vi "TOOLweb Rezept wechseln.vi"() -> ()   [LabVIEW 2020, in "FT-IR.lvlib" / "TOOLweb Interface.lvlib"]
doc: "Holt mit einer HTTP-POST-Anforderung gemäß TOOLweb-Protokoll Messdaten, Einstellungen und Diagnose-Information vom MKS MultiGas 2030 Analyzer. Alle Daten werden zeitsparend in einem einzigen Poll Request zusammengefasst, damit nur einmal eine TCP/IP-Verbindung geöffnet werden muss.\n\nAlle Ergebnis-Datentypen sind als Typdefinitionen in der Bibliothek \"Datentypen\" enthalten\" und erlauben so eine spätere Erweiterung.\n\nFalls \"Anzahl Gase\" unverbunden bleibt, wird der Standardwert 18 verwendet.\n \nFalls der TOOLWeb-Server nicht auf demselben Rechner arbeitet, kann mit \"IP-Adresse\" eine beliebiger Host adressiert werden. Ein unverbundener Eingang spricht den lokalen Host an."
uses:
  TOOLweb Interface.lvlib
  Aktion Rezeptwechsel.ctl
  Aktion FGV Rezepte wechseln.ctl
  Aktionen EVID-Codes.ctl
  Trigger Aktionen.ctl
  Sprachverwaltung/FGV Aktion Tabelle zerlegen.ctl
  Funktionstasten/Freigabe Aktionen.ctl
  FGV FT-IR Diagnose Aktionen.ctl
  SysLog/SysLog Interface.ctl
  FGV FT-IR Aktionen.ctl
  Erweiterte Konfig/Konfig CG-Check/Aktion Aenderung bei Rezeptwechsel.ctl
  AK-Schnittstelle/AK Namen Aktionen.ctl
  FGV FT-IR Gasliste Aktionen.ctl
  Messdaten/Aktionen FGV Messdaten.ctl
  EPA 1065/Allgemeine VIs/Aktion Wertaenderung Gasliste.ctl
  Bildwechsel/Bild-Auswahl.ctl
  FT-IR.lvlib
  Allgemein/allgemeine Sub-VIs.lvlib
  Funktionstasten/Funktionstasten.lvlib
  Messdaten/Messdaten.lvlib
  Log Konfig/LogKonfig.lvlib
  Typdefinitionen.lvlib
  Bildwechsel/Bildwechsel.lvlib
  Erweiterte Konfig/Konfig CG-Check/CG-Check Konfig.lvlib
  AK interface/AK-Interface.lvlib
  AK interface/Kommandos verwalten Aktionen.ctl
  SysLog/SysLog.lvlib
  Sprachverwaltung/Sprachverwaltung.lvlib
  EPA 1065/EPA 1065.lvlib
  AK-Schnittstelle/AK-Schnittstelle.lvlib
panel:
  out "Feedback":i32
  out "reject code":string
  out "Status Rezept":string
  out "Neues Rezept":string
  # "Rezeptwechsel wird durchgeführt"
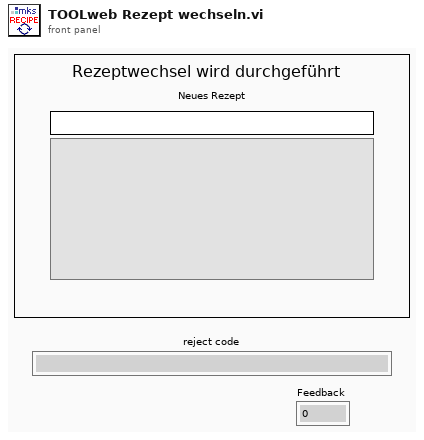
[diagram p1: front panel]
types:
  T1 = typedef "Sprachverwaltung.lvlib/FGV Aktion Tabelle zerlegen.ctl" = enum16{"laden", "vereinzeln", "speichern"}
  T2 = typedef "FT-IR.lvlib/TOOLweb Interface.lvlib/Typdefinitionen.lvlib/Trigger Aktionen.ctl" = enum16{"startrun", "runonce", "stoprun", "pauserun", "resumerun", "takeback"}
  T3 = typedef "FT-IR.lvlib/Aktionen EVID-Codes.ctl" = enum16{"lesen", "setzen", "laden", "speichern", "1Hz/5Hz", "Smoothing", "Rolling Average"}
  T4 = typedef "FT-IR.lvlib/Aktion FGV Rezepte wechseln.ctl" = enum16{"lesen", "Rezepte", "Rezeptindex", "Diesel", "Gasoline", "NCG", "laden", "speichern", "AK/Man"}
  T5 = typedef "FT-IR.lvlib/TOOLweb Interface.lvlib/Aktion Rezeptwechsel.ctl" = enum16{"Rezept wechsel", "Fehler", "Fehler 20", "Rezept geladen", "MG Bereit", "MG reagiert nicht", "Fertig", "Stoprun", "ueberpruefen"}
  T6 = typedef "Funktionstasten.lvlib/Freigabe Aktionen.ctl" = enum16{"prüfen", "Freigabe?", "lesen"}
  T7 = typedef "FT-IR.lvlib/AK-manuell.ctl" = enum16{"manuell", "Diesel", "CNG", "Gasoline"}
  T8 = typedef "FT-IR.lvlib/FGV FT-IR Diagnose Aktionen.ctl" = enum16{"Lesen", "Diagnose Schreiben", "Min Schreiben", "Max Schreiben"}
  T9 = cluster{"LaserPP Max":dbl, "LinCheck Max":dbl, "sBeam Max":dbl}
  T10 = cluster{"LaserPP Min":dbl, "LinCheck Min":dbl, "sBeam Min":dbl}
  T11 = typedef "FT-IR.lvlib/TOOLweb Interface.lvlib/Typdefinitionen.lvlib/TOOLweb Diagnose.ctl" = cluster{"(14) temperature":sgl, "(15) pressure":sgl, "(16) oxygen":sgl, "(50) diag-igramdc":sgl, "(51) diag-igrampp":sgl, "(52) diag-phaseAngle":sgl, "(53) diag-laserpp":sgl, "(54) diag-laserdc":sgl, "(55) diag-badscan":sgl, "(56) diag-centerburst":sgl, "(57) diag-linearizerCheck":sgl, "(58) diag-SNR":sgl, "(59) diag-sBeamIntensity":sgl}
  T12 = typedef "SysLog.lvlib/SysLog Interface.ctl" = cluster{"FehlermeldungsCode":i32, "ErfolgsmeldungsCode":i32, "ParameterListenString":string, "Anzeige":bool, "SysLogIcon":enum16{"OK", "Warnung", "Fehler"}, "intern":bool}
  T13 = typedef "FT-IR.lvlib/FGV FT-IR Aktionen.ctl" = enum16{"lesen", "NOG setzen", "NOS setzen", "Initialisieren", "speichern", "ALLES setzen", "FT-IR Spektrum loggen", "Komm Stoppen", "Spektrum LogKonfig"}
  T14 = typedef "AK-Schnittstelle.lvlib/AK Namen Aktionen.ctl" = enum16{"lesen", "laden", "speichern Namen", "AK Namen", "Liste erstellen", "EKFG erstellen", "speichern EKFG", "EKFG schreiben", "Neuen Eintrag erzeugen"}
  T15 = typedef "Erweiterte Konfig.lvlib/CG-Check Konfig.lvlib/Aktion Aenderung bei Rezeptwechsel.ctl" = enum16{"String erzeugen", "Index erzeugen"}
  T16 = typedef "FT-IR.lvlib/AK-Interface.lvlib/Kommandos verwalten Aktionen.ctl" = enum16{"lesen", "setzen Ende", "setzen Pos1", "senden", "initalisieren", "prüfen", "Kommandos"}
  T17 = typedef "FT-IR.lvlib/FGV FT-IR Gasliste Aktionen.ctl" = enum16{"lesen", "Gasliste FT-IR", "Gasliste ausgelesen", "laden", "speichern", "löschen"}
  T18 = typedef "Messdaten.lvlib/Aktionen FGV Messdaten.ctl" = enum16{"lesen", "schreiben", "löschen", "Mittelwerte", "Komponente"}
  T19 = typedef "EPA 1065.lvlib/Aktion Wertaenderung Gasliste.ctl" = enum16{"Init", "lesen", "Gasliste geändert", "ARN inaktiv", "LEAK inaktiv", "Interference 366 inaktiv", "T90 inaktiv", "Interference 375 inaktiv", "Chiller inaktiv", "FID O2 inaktiv", "FID Opti inaktiv", "Drift inaktiv", "Pre Test inaktiv", "LinV2 inaktiv"}
  T20 = typedef "Bildwechsel.lvlib/Bild-Auswahl.ctl" = enum16{"lesen", "Initialisieren", "Beenden", "Grafik", "Anlagenübersicht", "Anlagengrenzwerte", "Log Konfig", "Gaszuordnung AO", "Erw. Konfiguration", "FT-IR  ", "Störmeldungen", "Störmeldepuffer", "Störmeldekonfig", "PNS Grenzwerte", "Statusübersicht", "Linearisierung", "ARN", "EPA Dichtheitstest", "FID", "PMA", "CalGas", "Lambda", "Interference", "Amium PNS", "EPA T90", "Interference N2O", "Scheduler", "Systemeinstellungen", "EPA Drift", "CAN Konfig"}
  T21 = typedef "String - Ausgabefeld.ctl" = string
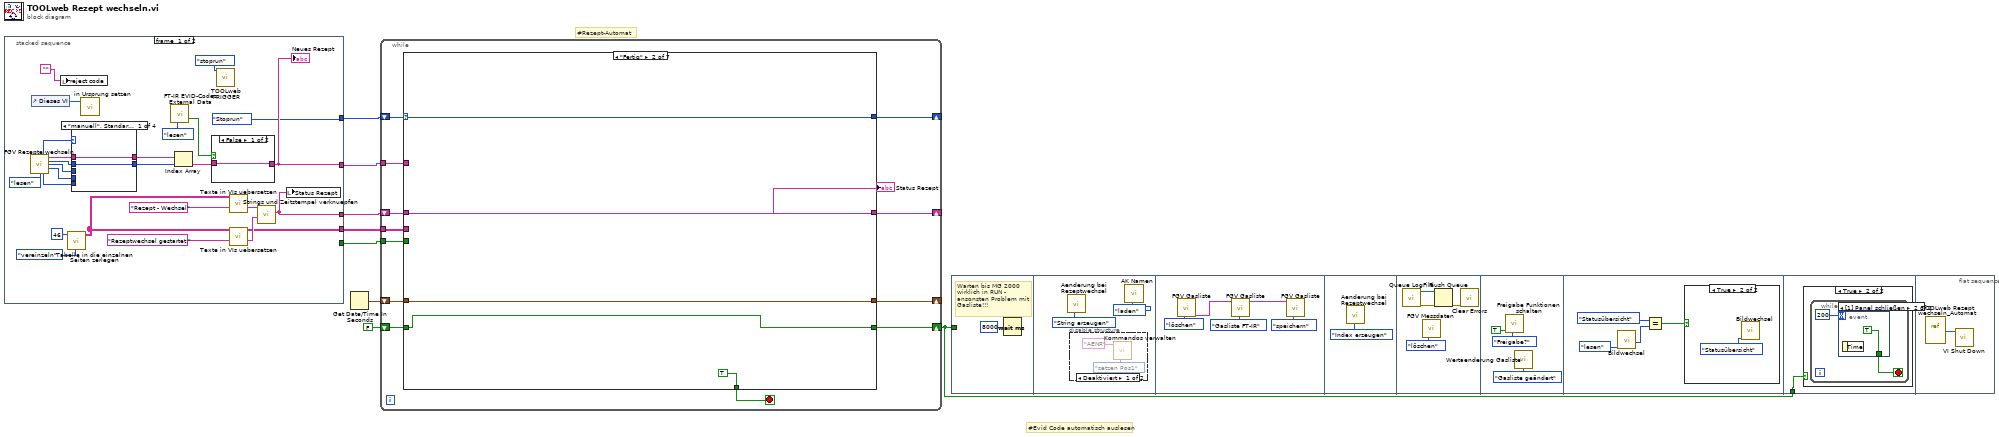
[diagram p0: block diagram]
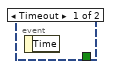
[diagram p5: hidden frame]
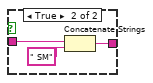
[diagram p6: hidden frame]
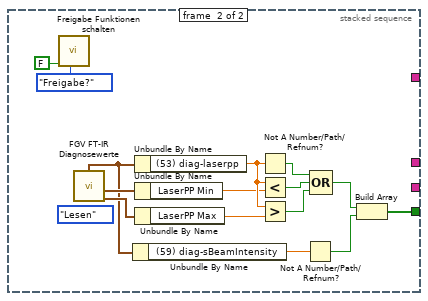
[diagram p10: hidden frame]
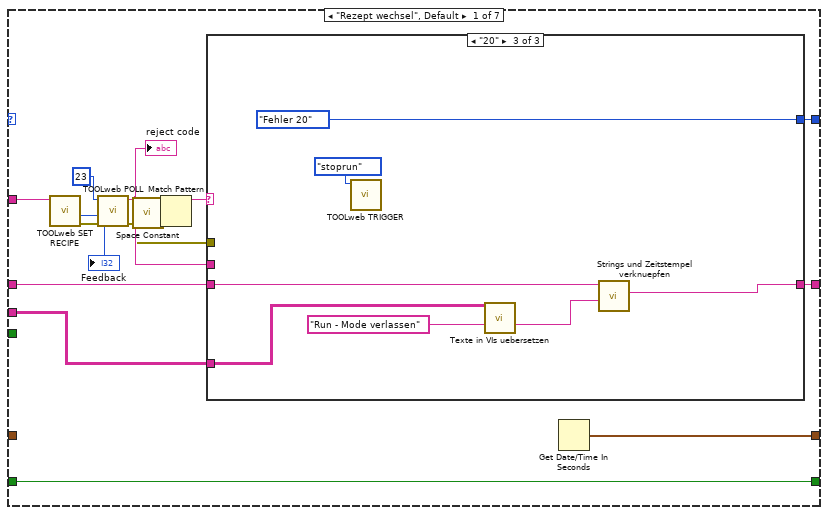
[diagram p11: hidden frame]
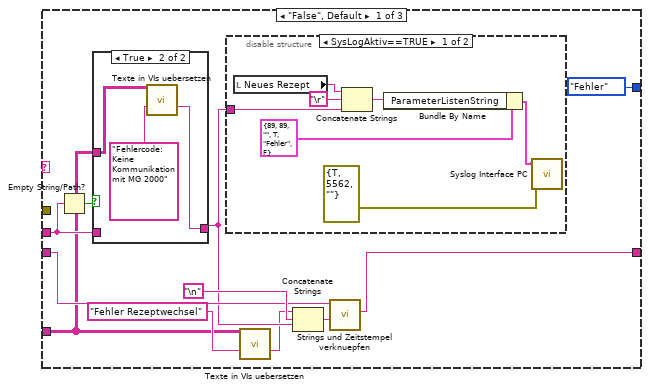
[diagram p12: hidden frame]
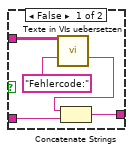
[diagram p14: hidden frame]
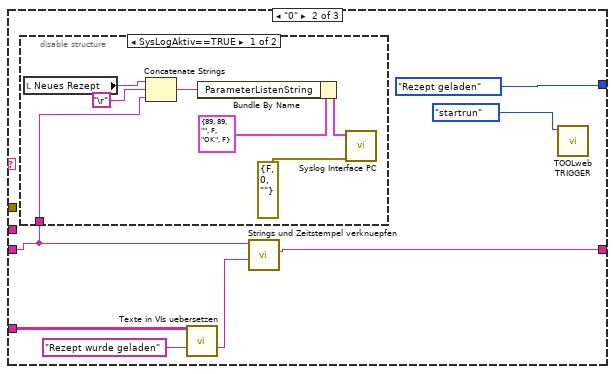
[diagram p15: hidden frame]
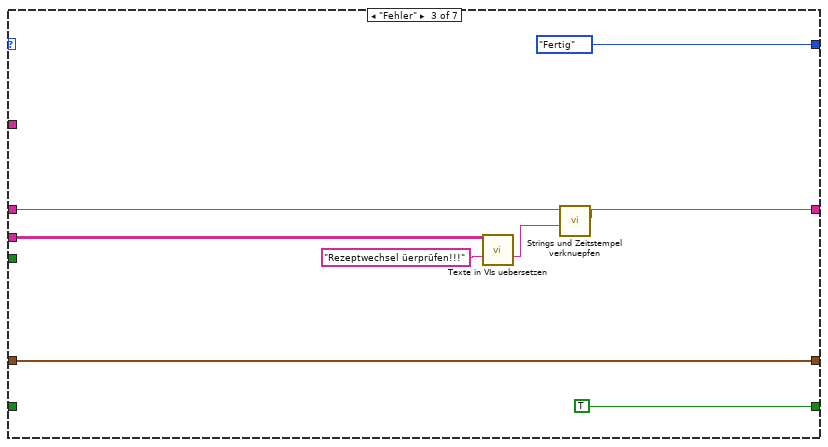
[diagram p17: hidden frame]
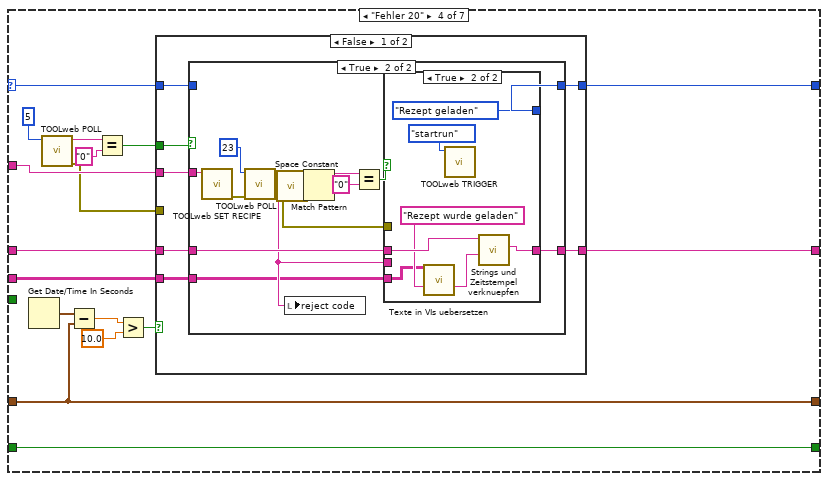
[diagram p18: hidden frame]
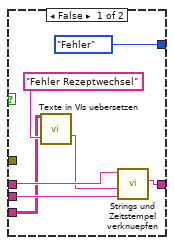
[diagram p20: hidden frame]
diagram:
  # "#Evid Code automatisch auslesen"
  # "#Rezept-Automat"
  n1 = stacked-sequence {
    tunnel: [w22 _] -> w8
    tunnel: [Aktion_Rezeptwechsel."Stoprun" ("Enum") _] -> w7
    tunnel: [w20 _] -> w6
    tunnel: [_ w47] -> w4
    tunnel: [w9 _] -> w1
    frame #0 {
      n2 = call "FGV Rezepte wechseln.vi"("Aktion"=Aktion_FGV_Rezepte_wechseln."lesen") -> ("AK/man"=w24:T7, "Rezepte"=w33:string[], "Rezeptindex"=w26:i32, "Diesel"=w28:u16, "Gasoline"=w29:u16, "Natural Gas"=w30:u16)  [unwired: 8 in, 1 out]
      n3 = control-ref of="Dieses VI"() -> (w18:refnum<vi>)
      n4 = local write "reject code"("") -> ()
      n5 = call "Tabelle in die einzelnen Seiten zerlegen.vi"("Aktion"=FGV_Aktion_Tabelle_zerlegen."vereinzeln", "Index (Seite)"=46) -> ("Sprachliste"=w10:string[][])  [unwired: 7 in, 2 out]
      n6 = case shown="\"manuell\", Standard" w24 {
        tunnel: w33 -> [w40 w42 w44 w45]
        tunnel: [w40 w42 w44 w45] -> w25
        tunnel: w26 -> [w39 _ _ _]
        tunnel: [w39 w41 w43 w46] -> w27
        tunnel: w28 -> [_ w41 _ _]
        tunnel: w29 -> [_ _ _ w46]
        tunnel: w30 -> [_ _ w43 _]
        frame "manuell", Default {
        }
        frame "Diesel" {
        }
        frame "CNG" {
        }
        frame "Gasoline" {
        }
      }
      n7 = call "in Ursprung setzen.vi"("VI Referenz"=w18) -> ()  [unwired: 10 in, 1 out]
      n8 = call "FT-IR EVID-Codes External Data.vi"("Aktionen"=Aktionen_EVID-Codes."lesen") -> ("Smoothing?"=w32:bool)  [unwired: 9 in, 5 out]
      n9 = Index Array(array=w25, index=w27) -> (element=w34:string)
      n10 = case shown="False" w32 {
        tunnel: w34 -> [w35 w37]
        tunnel: [w35 w38] -> w22
        frame False {
        }
        frame True {
          n11 = Concatenate Strings(w37, " SM" ("String")) -> (w38:string)
        }
      }
      "Neues Rezept" <- w22
      n12 = call "TOOLweb TRIGGER.vi"("action"=Trigger_Aktionen."stoprun") -> ()  [unwired: 5 in, 2 out]
      n13 = call "Texte in VIs uebersetzen.vi"("Sprachliste"=w10, "String zum Übersetzen"="Rezept - Wechsel") -> ("String zum Übersetzen"=w13:string)  [unwired: 9 in, 4 out]
      n14 = call "Texte in VIs uebersetzen.vi"("Sprachliste"=w10, "String zum Übersetzen"="Rezeptwechsel gestartet:") -> ("Sprachliste out"=w9:string[][], "String zum Übersetzen"=w11:string)  [unwired: 9 in, 3 out]
      n15 = call "Strings und Zeitstempel verknuepfen.vi"("String 1 hinzufügen"=w11, "Eingagns String"=w13) -> ("Verknüpfter String"=w20:string)  [unwired: 9 in]
      n16 = local write "Status Rezept"(w20) -> ()
    }
    frame #1 {
      (unwired) FGV_FT-IR_Diagnose_Aktionen."Lesen" ("Aktionen")
      n17 = call "Freigabe Funktionen schalten.vi"("Aktionen"=Freigabe_Aktionen."Freigabe?", "Freigabe?"=FALSE) -> ()  [unwired: 7 in, 3 out]
      n18 = call "FGV FT-IR Diagnosewerte.vi"() -> ("FT-IR MAX"=w58:T9, "FT-IR MIN"=w59:T10, "Diagnose"=w51:T11)  [unwired: 6 in, 3 out]
      n19 = Unbundle By Name(w51) -> ("(59) diag-sBeamIntensity"=w50:sgl)
      n20 = Unbundle By Name(w51) -> ("(53) diag-laserpp"=w57:sgl)
      n21 = Unbundle By Name(w59) -> ("LaserPP Min"=w56:dbl)
      n22 = Unbundle By Name(w58) -> ("LaserPP Max"=w55:dbl)
      n23 = Not A Number/Path/Refnum?(number/path/refnum=w57) -> (NaN/Path/Refnum?=w52:bool)
      n24 = Less?(x=w57, y=w56) -> (x < y?=w53:bool)
      n25 = Greater?(x=w57, y=w55) -> (0:w54:bool)
      n26 = Not A Number/Path/Refnum?(number/path/refnum=w50) -> (NaN/Path/Refnum?=w48:bool)
      n27 = Compound Arithmetic op=OR(w52, w53, w54) -> (w49:bool)
      n28 = Build Array(w49, w48) -> (w47:bool[])
    }
  }
  n29 = Get Date/Time In Seconds() -> (seconds since 1Jan1904=w2:timestamp)
  n30 = while {
    tunnel: w8 -> [w73]
    shift-right: [w72] -> _
    shift-left: w7 -> [w71]
    shift-right: [w70] -> _
    shift-left: w2 -> [w69]
    shift-right: [w65] -> _
    shift-left: w6 -> [w68]
    shift-right: [w66] -> w3
    shift-left: FALSE -> [w64]
    tunnel: w4 -> [w63]
    tunnel: w1 -> [w62]
    stop <- w67 stop-if-true
    n31 = case shown="\"Fertig\"" w71 {
      selector: w71 -> [_ w137 _ w153 w246 w285 _]
      tunnel: w73 -> [w87 _ _ w152 w245 w274 _]
      tunnel: [w82 w137 Aktion_Rezeptwechsel."Fertig" ("Enum") w160 w253 w286 Aktion_Rezeptwechsel."Fehler" ("Enum")] -> w72
      tunnel: w69 -> [_ w139 w146 w151 w244 w294 w329]
      tunnel: [w78 w139 w146 w151 w244 w294 w329] -> w70
      tunnel: w68 -> [w81 w138 w143 w159 w252 w282 w326]
      tunnel: [w80 w138 w144 w154 w247 w283 w328] -> w65
      tunnel: [_ TRUE _ _ _ _ _] -> w67
      tunnel: [w76 w135 TRUE w150 w243 w277 w327] -> w66
      tunnel: w64 -> [w76 w135 _ w150 w243 w277 w327]
      tunnel: w63 -> [_ _ _ _ _ _ _]
      tunnel: w62 -> [w74 _ w140 w148 _ w270 w323]
      frame "Rezept wechsel", Default {
        n32 = call "TOOLweb SET RECIPE.vi"("Recipe Name"=w87) -> ("error out"=w85:errorcluster, "Feedback"=→"Feedback":i32)  [unwired: 4 in, 1 out]
        n33 = call "TOOLweb POLL.vi"("error in (no error)"=w85, "EVID-Nummer"=23) -> ("error out"=w75:errorcluster, "Wert-String"=w79:string)  [unwired: 4 in]
        "reject code" <- w79
        n34 = call <vilib>:"Space Constant.vi"() -> ("String"=w84:string)
        n35 = Match Pattern(string=w79, regular expression=w84) -> (before substring=w83:string)  [unwired: 1 in, 3 out]
        n36 = case shown="\"20\"" w83 {
          tunnel: [Aktion_Rezeptwechsel."Fehler" ("Enum") Aktion_Rezeptwechsel."Rezept geladen" ("Enum") Aktion_Rezeptwechsel."Fehler 20" ("Enum")] -> w82
          tunnel: w81 -> [w95 w117 w131]
          tunnel: [w94 w119 w132] -> w80
          tunnel: w79 -> [w92 _ _]
          tunnel: w75 -> [_ _ _]
          tunnel: w74 -> [w88 w114 w128]
          frame "False", Default {
            n37 = Empty String/Path?(string/path=w92) -> (empty?=w93:bool)
            n38 = case shown="True" w93 {
              tunnel: [w110 w112] -> w91
              tunnel: w92 -> [w109 _]
              tunnel: w88 -> [w106 w111]
              frame False {
                n39 = call "Texte in VIs uebersetzen.vi"("Sprachliste"=w106, "String zum Übersetzen"="Fehlercode:" ("String")) -> ("String zum Übersetzen"=w107:string)  [unwired: 9 in, 4 out]
                n40 = Concatenate Strings(w107, w109) -> (w110:string)
              }
              frame True {
                n41 = call "Texte in VIs uebersetzen.vi"("Sprachliste"=w111, "String zum Übersetzen"="Fehlercode: Keine Kommunikation mit MG 2000" ("String")) -> ("String zum Übersetzen"=w112:string)  [unwired: 9 in, 4 out]
              }
            }
            n42 = disable-structure shown="SysLogAktiv==TRUE" {
              disable-tunnel: w91 -> [w102 _]
              frame condition #0 (active) {
                n43 = local read "Neues Rezept"() -> (w104:string)
                n44 = Concatenate Strings(w104, "\r", w102) -> (w99:string)
                n45 = Bundle By Name(cluster=T12 {"FehlermeldungsCode"=89, "ErfolgsmeldungsCode"=89, "ParameterListenString"="", "Anzeige"=TRUE, "SysLogIcon"=enum."Fehler", "intern"=FALSE} ("Cluster (in)"), "ParameterListenString"=w99) -> (w100:T12)
                n46 = call "Syslog Interface PC.vi"("Fehler (in)"=errorcluster {"status"=TRUE, "code"=5562, "source"=""}, "Cluster (in)"=w100) -> ()  [unwired: 9 in, 1 out]
              }
              frame condition #1 {
              }
            }
            n47 = call "Texte in VIs uebersetzen.vi"("Sprachliste"=w88, "String zum Übersetzen"="Fehler Rezeptwechsel" ("String")) -> ("String zum Übersetzen"=w89:string)  [unwired: 9 in, 4 out]
            n48 = Concatenate Strings(w89, "\n", w91) -> (w96:string)
            n49 = call "Strings und Zeitstempel verknuepfen.vi"("String 1 hinzufügen"=w96, "Eingagns String"=w95) -> ("Verknüpfter String"=w94:string)  [unwired: 9 in]
          }
          frame "0" {
            n50 = disable-structure shown="SysLogAktiv==TRUE" {
              disable-tunnel: w117 -> [w124 _]
              frame condition #0 (active) {
                n51 = local read "Neues Rezept"() -> (w126:string)
                n52 = Concatenate Strings(w126, "\r", w124) -> (w121:string)
                n53 = Bundle By Name(cluster=T12 {"FehlermeldungsCode"=89, "ErfolgsmeldungsCode"=89, "ParameterListenString"="", "Anzeige"=FALSE, "SysLogIcon"=enum."OK", "intern"=FALSE} ("Cluster (in)"), "ParameterListenString"=w121) -> (w122:T12)
                n54 = call "Syslog Interface PC.vi"("Fehler (in)"=errorcluster {"status"=FALSE, "code"=0, "source"=""}, "Cluster (in)"=w122) -> ()  [unwired: 9 in, 1 out]
              }
              frame condition #1 {
              }
            }
            n55 = call "Texte in VIs uebersetzen.vi"("Sprachliste"=w114, "String zum Übersetzen"="Rezept wurde geladen" ("String")) -> ("String zum Übersetzen"=w115:string)  [unwired: 9 in, 4 out]
            n56 = call "Strings und Zeitstempel verknuepfen.vi"("String 1 hinzufügen"=w115, "Eingagns String"=w117) -> ("Verknüpfter String"=w119:string)  [unwired: 9 in]
            n57 = call "TOOLweb TRIGGER.vi"("action"=Trigger_Aktionen."startrun") -> ()  [unwired: 5 in, 2 out]
          }
          frame "20" {
            n58 = call "TOOLweb TRIGGER.vi"("action"=Trigger_Aktionen."stoprun") -> ()  [unwired: 5 in, 2 out]
            n59 = call "Texte in VIs uebersetzen.vi"("Sprachliste"=w128, "String zum Übersetzen"="Run - Mode verlassen" ("String")) -> ("String zum Übersetzen"=w129:string)  [unwired: 9 in, 4 out]
            n60 = call "Strings und Zeitstempel verknuepfen.vi"("String 1 hinzufügen"=w129, "Eingagns String"=w131) -> ("Verknüpfter String"=w132:string)  [unwired: 9 in]
          }
        }
        n61 = Get Date/Time In Seconds() -> (seconds since 1Jan1904=w78:timestamp)
      }
      frame "Fertig" {
      }
      frame "Fehler" {
        n62 = call "Texte in VIs uebersetzen.vi"("Sprachliste"=w140, "String zum Übersetzen"="Rezeptwechsel üerprüfen!!!" ("String")) -> ("String zum Übersetzen"=w141:string)  [unwired: 9 in, 4 out]
        n63 = call "Strings und Zeitstempel verknuepfen.vi"("String 1 hinzufügen"=w141, "Eingagns String"=w143) -> ("Verknüpfter String"=w144:string)  [unwired: 9 in]
      }
      frame "Fehler 20" {
        n64 = Get Date/Time In Seconds() -> (seconds since 1Jan1904=w164:timestamp)
        n65 = call "TOOLweb POLL.vi"("EVID-Nummer"=5) -> ("error out"=w149:errorcluster, "Wert-String"=w157:string)  [unwired: 5 in]
        n66 = Subtract(x=w164, y=w151) -> (x-y=w163:dbl)
        n67 = Equal?(x=w157, y="0") -> (x = y?=w155:bool)
        n68 = Greater?(x=w163, y=10.0) -> (0:w161:bool)
        n69 = case shown="False" w161 {
          tunnel: [w170 w206] -> w160
          tunnel: w159 -> [w167 w204]
          tunnel: w155 -> [w171 w202]
          tunnel: [w168 w205] -> w154
          tunnel: w153 -> [w169 _]
          tunnel: w152 -> [w166 w203]
          tunnel: w149 -> [_ _]
          tunnel: w148 -> [w165 w201]
          frame False {
            n70 = case shown="True" w171 {
              tunnel: [w173 w179] -> w170
              tunnel: w169 -> [w173 _]
              tunnel: [w172 w177] -> w168
              tunnel: w167 -> [w172 w178]
              tunnel: w166 -> [_ w186]
              tunnel: w165 -> [_ w174]
              frame False {
              }
              frame True {
                n71 = call "TOOLweb SET RECIPE.vi"("Recipe Name"=w186) -> ("error out"=w183:errorcluster)  [unwired: 4 in, 2 out]
                n72 = call "TOOLweb POLL.vi"("error in (no error)"=w183, "EVID-Nummer"=23) -> ("error out"=w175:errorcluster, "Wert-String"=w176:string)  [unwired: 4 in]
                n73 = call <vilib>:"Space Constant.vi"() -> ("String"=w184:string)
                n74 = local write "reject code"(w176) -> ()
                n75 = Match Pattern(string=w176, regular expression=w184) -> (before substring=w182:string)  [unwired: 1 in, 3 out]
                n76 = Equal?(x=w182, y="0") -> (x = y?=w180:bool)
                n77 = case shown="True" w180 {
                  tunnel: [Aktion_Rezeptwechsel."Fehler" ("Enum") Aktion_Rezeptwechsel."Rezept geladen" ("Enum")] -> w179
                  tunnel: w178 -> [w192 w198]
                  tunnel: [w190 w197] -> w177
                  tunnel: w176 -> [w191 _]
                  tunnel: w175 -> [_ _]
                  tunnel: w174 -> [w187 w194]
                  frame False {
                    n78 = call "Texte in VIs uebersetzen.vi"("Sprachliste"=w187, "String zum Übersetzen"="Fehler Rezeptwechsel" ("String")) -> ("String zum Übersetzen"=w188:string)  [unwired: 9 in, 4 out]
                    n79 = call "Strings und Zeitstempel verknuepfen.vi"("String 2 hinzufügen"=w191, "String 1 hinzufügen"=w188, "Eingagns String"=w192) -> ("Verknüpfter String"=w190:string)  [unwired: 8 in]
                  }
                  frame True {
                    n80 = call "Texte in VIs uebersetzen.vi"("Sprachliste"=w194, "String zum Übersetzen"="Rezept wurde geladen" ("String")) -> ("String zum Übersetzen"=w195:string)  [unwired: 9 in, 4 out]
                    n81 = call "TOOLweb TRIGGER.vi"("action"=Trigger_Aktionen."startrun") -> ()  [unwired: 5 in, 2 out]
                    n82 = call "Strings und Zeitstempel verknuepfen.vi"("String 1 hinzufügen"=w195, "Eingagns String"=w198) -> ("Verknüpfter String"=w197:string)  [unwired: 9 in]
                  }
                }
              }
            }
          }
          frame True {
            n83 = disable-structure shown="Aktiviert" {
              disable-tunnel: [Aktion_Rezeptwechsel."MG reagiert nicht" ("Enum") w216] -> w206
              disable-tunnel: [w209 w215] -> w205
              disable-tunnel: w204 -> [w208 w214]
              disable-tunnel: w203 -> [_ w213]
              disable-tunnel: w202 -> [_ w212]
              disable-tunnel: w201 -> [_ w211]
              frame Disabled {
                n84 = call "Strings und Zeitstempel verknuepfen.vi"("String 1 hinzufügen"="MG 2000 reagiert nicht" ("String"), "Eingagns String"=w208) -> ("Verknüpfter String"=w209:string)  [unwired: 9 in]
              }
              frame Enabled {
                n85 = case shown="True" w212 {
                  tunnel: [Aktion_Rezeptwechsel."Fehler" ("Enum") Aktion_Rezeptwechsel."Rezept geladen" ("Enum")] -> w216
                  tunnel: w213 -> [w221 w240]
                  tunnel: [w220 w239] -> w215
                  tunnel: w214 -> [w222 _]
                  tunnel: w211 -> [w217 w236]
                  frame False {
                    n86 = Empty String/Path?(string/path=w221) -> (empty?=w224:bool)
                    n87 = case shown="False" w224 {
                      tunnel: [w232 w234] -> w225
                      tunnel: w221 -> [w231 _]
                      tunnel: w217 -> [w228 w233]
                      frame False {
                        n88 = call "Texte in VIs uebersetzen.vi"("Sprachliste"=w228, "String zum Übersetzen"="Fehlercode:" ("String")) -> ("String zum Übersetzen"=w229:string)  [unwired: 9 in, 4 out]
                        n89 = Concatenate Strings(w229, w231) -> (w232:string)
                      }
                      frame True {
                        n90 = call "Texte in VIs uebersetzen.vi"("Sprachliste"=w233, "String zum Übersetzen"="Fehlercode: Keine Kommunikation mit MG 2000" ("String")) -> ("String zum Übersetzen"=w234:string)  [unwired: 9 in, 4 out]
                      }
                    }
                    n91 = call "Texte in VIs uebersetzen.vi"("Sprachliste"=w217, "String zum Übersetzen"="Fehler Rezeptwechsel" ("String")) -> ("String zum Übersetzen"=w218:string)  [unwired: 9 in, 4 out]
                    n92 = Concatenate Strings(w218, "\n", w225) -> (w226:string)
                    n93 = call "Strings und Zeitstempel verknuepfen.vi"("String 1 hinzufügen"=w226, "Eingagns String"=w222) -> ("Verknüpfter String"=w220:string)  [unwired: 9 in]
                  }
                  frame True {
                    n94 = call "Texte in VIs uebersetzen.vi"("Sprachliste"=w236, "String zum Übersetzen"="Rezept wurde geladen" ("String")) -> ("String zum Übersetzen"=w237:string)  [unwired: 9 in, 4 out]
                    n95 = call "Strings und Zeitstempel verknuepfen.vi"("String 1 hinzufügen"=w237, "Eingagns String"=w240) -> ("Verknüpfter String"=w239:string)  [unwired: 9 in]
                  }
                }
              }
            }
          }
        }
      }
      frame "Stoprun" {
        n96 = Get Date/Time In Seconds() -> (seconds since 1Jan1904=w257:timestamp)
        n97 = call "TOOLweb POLL.vi"("EVID-Nummer"=5) -> ("error out"=w242:errorcluster, "Wert-String"=w250:string)  [unwired: 5 in]
        n98 = Subtract(x=w257, y=w244) -> (x-y=w256:dbl)
        n99 = call <vilib>:"Clear Errors.vi"("error in (no error)"=w242) -> ()  [unwired: 5 in, 2 out]
        n100 = Equal?(x=w250, y="0") -> (x = y?=w248:bool)
        n101 = Greater?(x=w256, y=10.0) -> (0:w254:bool)
        n102 = case shown="False" w254 {
          tunnel: [w262 Aktion_Rezeptwechsel."Rezept wechsel" ("Enum")] -> w253
          tunnel: w252 -> [w259 w268]
          tunnel: w248 -> [w263 _]
          tunnel: [w260 w268] -> w247
          tunnel: w246 -> [w261 _]
          tunnel: w245 -> [w258 _]
          frame False {
            n103 = case shown="False" w263 {
              tunnel: [w265 Aktion_Rezeptwechsel."Rezept wechsel" ("Enum")] -> w262
              tunnel: w261 -> [w265 _]
              tunnel: [w264 w266] -> w260
              tunnel: w259 -> [w264 w266]
              tunnel: w258 -> [_ _]
              frame False {
              }
              frame True {
              }
            }
          }
          frame True {
          }
        }
      }
      frame "Rezept geladen" {
        n104 = Get Date/Time In Seconds() -> (seconds since 1Jan1904=w297:timestamp)
        n105 = call "TOOLweb POLL.vi"("EVID-Nummer"=53) -> ("error out"=w272:errorcluster, "Wert-String"=w290:string)  [unwired: 5 in]
        n106 = call "TOOLweb POLL.vi"("EVID-Nummer"=5) -> ("error out"=w271:errorcluster, "Wert-String"=w292:string)  [unwired: 5 in]
        n107 = call "FGV FT-IR Parameter.vi"("Aktion"=FGV_FT-IR_Aktionen."lesen") -> ("Current Recipe"=w275:string)  [unwired: 11 in, 7 out]
        n108 = Subtract(x=w297, y=w294) -> (x-y=w296:dbl)
        n109 = Fract/Exp String To Number(string=w290) -> (offset past number=w278:i32)  [unwired: 3 in, 1 out]
        n110 = Equal?(x=w292, y="2") -> (x = y?=w281:bool)
        n111 = Equal?(x=w274, y=w275) -> (x = y?=w273:bool)
        n112 = Greater?(x=w296, y=10.0) -> (0:w284:bool)
        n113 = In Range and Coerce(upper limit=12 ("x"), x=w278, lower limit=0 ("y")) -> (In Range?=w288:bool)  [unwired: 1 out]
        n114 = Compound Arithmetic op=AND ("Mehrfacharithmetik")(w281, w288, w273) -> (w287:bool)
        n115 = case shown="True" w284 {
          tunnel: w287 -> [w304 _]
          tunnel: [w303 Aktion_Rezeptwechsel."MG reagiert nicht" ("Enum")] -> w286
          tunnel: w285 -> [w302 _]
          tunnel: [w301 w322] -> w283
          tunnel: w282 -> [w300 w321]
          tunnel: w281 -> [w299 _]
          tunnel: w272 -> [_ _]
          tunnel: w271 -> [_ _]
          tunnel: w270 -> [w298 w317]
          frame False {
            n116 = case shown="False" w304 {
              tunnel: [w307 Aktion_Rezeptwechsel."Fertig" ("Enum")] -> w303
              tunnel: w302 -> [w307 _]
              tunnel: [w306 w313] -> w301
              tunnel: w300 -> [w306 w315]
              tunnel: w299 -> [w305 _]
              tunnel: w298 -> [_ w308]
              frame False {
                n117 = case shown="False" w305 {
                  frame False {
                    n118 = disable-structure shown="Aktiviert" {
                      frame Disabled {
                        (unwired) Trigger_Aktionen."startrun" ("action")
                        n119 = call "TOOLweb TRIGGER.vi"() -> ()  [unwired: 6 in, 2 out]
                      }
                      frame Enabled {
                      }
                    }
                  }
                  frame True {
                  }
                }
              }
              frame True {
                n120 = call "Texte in VIs uebersetzen.vi"("Sprachliste"=w308, "String zum Übersetzen"="MG 2000 bereit!" ("String")) -> ("String zum Übersetzen"=w311:string)  [unwired: 9 in, 4 out]
                n121 = call "Strings und Zeitstempel verknuepfen.vi"("String 1 hinzufügen"=w311, "Eingagns String"=w315) -> ("Verknüpfter String"=w314:string)  [unwired: 9 in]
                n122 = call "Texte in VIs uebersetzen.vi"("Sprachliste"=w308, "String zum Übersetzen"="Starten" ("String 2 hinzufügen")) -> ("String zum Übersetzen"=w309:string)  [unwired: 9 in, 4 out]
                n123 = call "Strings und Zeitstempel verknuepfen.vi"("String 1 hinzufügen"=w309, "Eingagns String"=w314) -> ("Verknüpfter String"=w313:string)  [unwired: 9 in]
              }
            }
          }
          frame True {
            n124 = call "Texte in VIs uebersetzen.vi"("Sprachliste"=w317, "String zum Übersetzen"="MG 2000 befindet\nsich nicht im Run - Mode!" ("String")) -> ("String zum Übersetzen"=w318:string)  [unwired: 9 in, 4 out]
            n125 = call "Strings und Zeitstempel verknuepfen.vi"("String 1 hinzufügen"=w318, "Eingagns String"=w321) -> ("Verknüpfter String"=w322:string)  [unwired: 9 in]
          }
        }
      }
      frame "MG reagiert nicht" {
        n126 = call "Texte in VIs uebersetzen.vi"("Sprachliste"=w323, "String zum Übersetzen"="MG reagiert nicht!" ("String")) -> ("String zum Übersetzen"=w324:string)  [unwired: 9 in, 4 out]
        n127 = call "Strings und Zeitstempel verknuepfen.vi"("String 1 hinzufügen"=w324, "Eingagns String"=w326) -> ("Verknüpfter String"=w328:string)  [unwired: 9 in]
      }
    }
    "Status Rezept" <- w65
  }
  n128 = flat-sequence {
    tunnel: w3 -> [_]
    tunnel: w3 -> [w354]
    frame #0 {
      # "Warten bis MG 2000\nwirklich in RUN - \nansonsten Problem mit \nGasliste!!!"
      n129 = Wait (ms)(milliseconds to wait=u32 8000 ("Zu wartende ms")) -> ()  [unwired: 1 out]
    }
    frame #1 {
      n130 = call "Aenderung bei Rezeptwechsel.vi"("Enum"=Aktion_Aenderung_bei_Rezeptwechsel."String erzeugen") -> ()  [unwired: 10 in, 1 out]
      n131 = disable-structure shown="Deaktiviert" {
        frame Disabled {
          n132 = call "Kommandos verwalten.vi"("Aktionen"=Kommandos_verwalten_Aktionen."setzen Pos1", "neues Kommando"="AENR") -> ()  [unwired: 7 in, 3 out]
        }
        frame Enabled {
        }
      }
      n133 = call "AK Namen.vi"("Aktionen"=AK_Namen_Aktionen."laden") -> ()  [unwired: 7 in, 4 out]
    }
    frame #2 {
      n134 = call "FGV Gasliste.vi"("Aktionen"=FGV_FT-IR_Gasliste_Aktionen."löschen") -> ("Gasliste ausgelesen"=w340:T21[])  [unwired: 8 in, 2 out]
      n135 = call "FGV Gasliste.vi"("Aktionen"=FGV_FT-IR_Gasliste_Aktionen."Gasliste FT-IR", "Aktuelle Gasliste FT-IR"=w340) -> ("Aktuelle Gasliste FT-IR"=w338:T21[])  [unwired: 7 in, 2 out]
      n136 = call "FGV Gasliste.vi"("Aktionen"=FGV_FT-IR_Gasliste_Aktionen."speichern", "Aktuelle Gasliste FT-IR"=w338) -> ()  [unwired: 7 in, 3 out]
    }
    frame #3 {
      n137 = call "Aenderung bei Rezeptwechsel.vi"("Enum"=Aktion_Aenderung_bei_Rezeptwechsel."Index erzeugen") -> ()  [unwired: 10 in, 1 out]
    }
    frame #4 {
      n138 = call "Queue LogFile.vi"() -> ("error out"=w342:errorcluster, "Queue (Ausgang)"=w343:refnum<queue>)  [unwired: 6 in]
      n139 = call "FGV Messdaten.vi"("Aktionen"=Aktionen_FGV_Messdaten."löschen") -> ()  [unwired: 6 in, 9 out]
      n140 = Flush Queue(queue=w343, error in (no error)=w342) -> (error out=w345:errorcluster)  [unwired: 2 out]
      n141 = call <vilib>:"Clear Errors.vi"("error in (no error)"=w345) -> ()  [unwired: 5 in, 2 out]
    }
    frame #5 {
      n142 = call "Freigabe Funktionen schalten.vi"("Aktionen"=Freigabe_Aktionen."Freigabe?", "Freigabe?"=TRUE) -> ()  [unwired: 7 in, 3 out]
      n143 = call "Wertaenderung Gasliste.vi"("Aktion"=Aktion_Wertaenderung_Gasliste."Gasliste geändert") -> ()  [unwired: 13 in, 2 out]
    }
    frame #6 {
      n144 = call "Bildwechsel.vi"("nächstes Bild"=Bild-Auswahl."lesen") -> ("aktuelle Bildnummer"=w351:T20)  [unwired: 3 in, 7 out]
      n145 = Equal?(x=Bild-Auswahl."Statusübersicht", y=w351) -> (x = y?=w349:bool)
      n146 = case shown="True" w349 {
        frame False {
        }
        frame True {
          n147 = call "Bildwechsel.vi"("nächstes Bild"=Bild-Auswahl."Statusübersicht") -> ()  [unwired: 3 in, 8 out]
        }
      }
    }
    frame #7 {
      n148 = case shown="True" w354 {
        frame False {
        }
        frame True {
          n149 = while {
            stop <- w355 stop-if-true
            n150 = event shown="[1] Panel schließen" {
              selector: _ -> [_ _]
              dyn-events: _ -> [_ _]
              timeout: 200 -> [_ _]
              tunnel: [_ TRUE] -> w355
              event Timeout {
                n151 = event-data() -> ()  [unwired: 1 in, 1 out]
              }
              event Panel Close {
                n152 = event-data() -> ()  [unwired: 1 in, 1 out]
              }
            }
          }
        }
      }
    }
    frame #8 {
      n153 = vi-ref "TOOLweb Rezept wechseln_Automat.vi"() -> (w358:refnum<vi>)
      n154 = call "VI Shut Down.vi"("VI Referenz"=w358) -> ()  [unwired: 11 in]
    }
  }
